vi "SERIAL_ValidateChecksum.vi"(1 "Expected Packet Length":i32, 2 "Content":string) -> (0 "Valid?":bool)   [LabVIEW 2014, in "navX-MXP IMU.lvlib"]
uses:
  navX-MXP IMU.lvlib
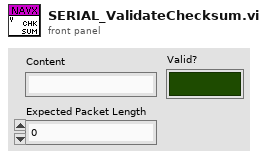
[diagram p1: front panel]
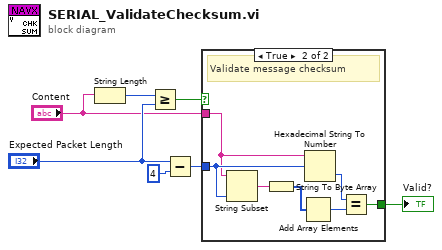
[diagram p0: block diagram]
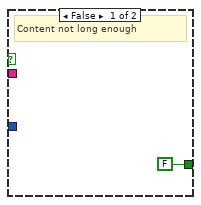
[diagram p2: hidden frame]
diagram:
  n1 = String Length(string="Content") -> (length=w7:i32)
  n2 = Greater Or Equal?(x=w7, y="Expected Packet Length") -> (x >= y?=w6:bool)
  n3 = Subtract(x="Expected Packet Length", y=4) -> (x-y=w2:i32)
  n4 = case shown="True" w6 {
    tunnel: [FALSE w10] -> w5
    tunnel: w2 -> [_ w15]
    tunnel: "Content" -> [_ w9]
    frame False {
      # "Content not long enough"
    }
    frame True {
      # "Validate message checksum"
      n5 = String Subset(string=w9, length (rest)=w15) -> (substring=w14:string)  [unwired: 1 in]
      n6 = String To Byte Array(string=w14) -> (unsigned byte array=w13:u8[])
      n7 = Add Array Elements(numeric array=w13) -> (sum=w11:u8)
      n8 = Hexadecimal String To Number(string=w9, offset=w15) -> (number=w12:u32)  [unwired: 1 in, 1 out]
      n9 = Equal?(x=w12, y=w11) -> (x = y?=w10:bool)
    }
  }
  "Valid?" <- w5
